vi "Analyze Acceleration (RT).vi"(9 "Max Instantaneous Acceleration (g)":sgl, 11 "Acceleration Waveform (SGL)":sgl[](array[numeric])) -> (1 "Over Limit?":bool, 2 "Acceleration (grms)":dbl, 3 "Acceleration Waveform (DBL)":dbl[](array[numeric]))   [LabVIEW 2017]
uses:
  <vilib>/Analysis/5stat.llb/RMS (DBL).vi
  <vilib>/Analysis/NI_AALPro.lvlib
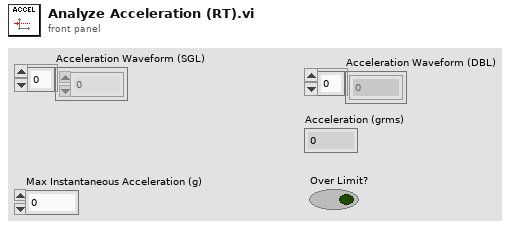
[diagram p1: front panel]
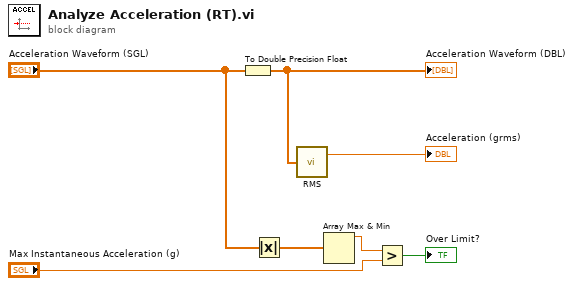
[diagram p0: block diagram]
diagram:
  n1 = To Double Precision Float(number="Acceleration Waveform (SGL)") -> (double precision float=w3:dbl[])
  "Acceleration Waveform (DBL)" <- w3
  n2 = Absolute Value(x="Acceleration Waveform (SGL)") -> (abs(x)=w5:sgl[])
  n3 = call-poly <vilib>:"RMS.vi"("X"=w3) -> ("rms value"=→"Acceleration (grms)":dbl)  [unwired: 1 out]
  n4 = Array Max & Min(array=w5) -> (max value=w6:sgl)  [unwired: 3 out]
  n5 = Greater?(x=w6, y="Max Instantaneous Acceleration (g)") -> (0:→"Over Limit?":bool)
